vi "Add event name to list.vi"(0 "Event Number":dbl, 1 "Event Name":string, 2 "file path (dialog if empty)":path) -> ()   [LabVIEW 2014]
uses:
  <vilib>/Utility/file.llb/Read From Spreadsheet File (string).vi
  <vilib>/Utility/file.llb/Write To Spreadsheet File (string).vi
panel:
  out "output array":string[](array[string])
  out "subarray":string[][](array[string])
  out "first row":string[](array[string])
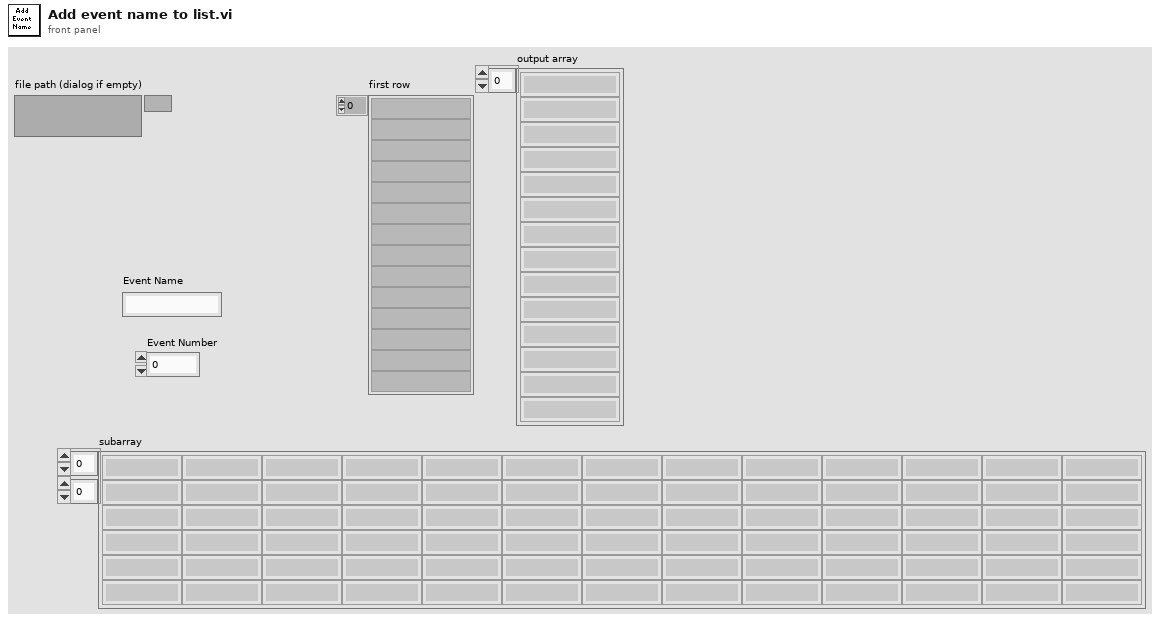
[diagram p1: front panel]
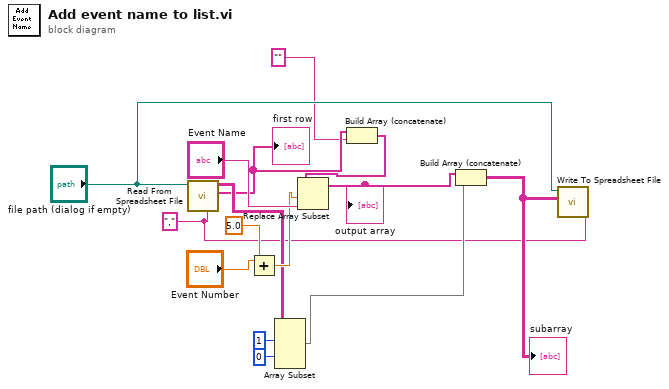
[diagram p0: block diagram]
diagram:
  w4 = "," ("delimiter (\\t)")
  n1 = call-poly <vilib>:"Read From Spreadsheet File.vi"("delimiter (\\t)"=w4, "file path (dialog if empty)"="file path (dialog if empty)") -> ("first row"=w3:string[], "all rows"=w11:string[][])  [unwired: 5 in, 3 out]
  "first row" <- w3
  n2 = Add(x="Event Number", y=5.0) -> (x+y=w14:dbl)
  n3 = Array Subset(array=w11, index (row)=1 ("index"), index (col)=0 ("index")) -> (w7:string[][])  [unwired: 2 in]
  n4 = Build Array (concatenate)(w3, "" ("delimiter (\\t)")) -> (w1:string[])
  n5 = Replace Array Subset(array=w1, new element="Event Name", index=w14) -> (w8:string[])
  "output array" <- w8
  n6 = Build Array (concatenate)(w8, w7) -> (w5:string[][])
  "subarray" <- w5
  n7 = call-poly <vilib>:"Write To Spreadsheet File.vi"("delimiter (\\t)"=w4, "2D data"=w5, "file path (dialog if empty)"="file path (dialog if empty)") -> ()  [unwired: 5 in, 1 out]
